vi "AAL Resample (const to Variable, complex single-channel).vi"(7 "reset? (True)":bool=TRUE, 8 "error in (no error)":errorcluster, 9 "config":T1={"timing jitter"=enum."Interpolation", "anti-aliasing?"=TRUE, "filter prototype"={"coefficients"=[], "factor"=1}} {"filter prototype"."coefficients" format="%.2f"}, 10 "time":dbl[](array[numeric]) format="%.2f", 11 "X":cdb[](array[numeric])) -> (0 "error out":errorcluster, 1 "offset":i64, 2 "time stamps":dbl[](array[numeric]) format="%.2f", 3 "Y":cdb[](array[numeric]) format="%.2f")   [LabVIEW 2017, in "NI_AALPro.lvlib"]
doc: "Perform an arbitrary resampling on the input signal."
uses:
  NI_AALPro.lvlib
  lvanlys.dll
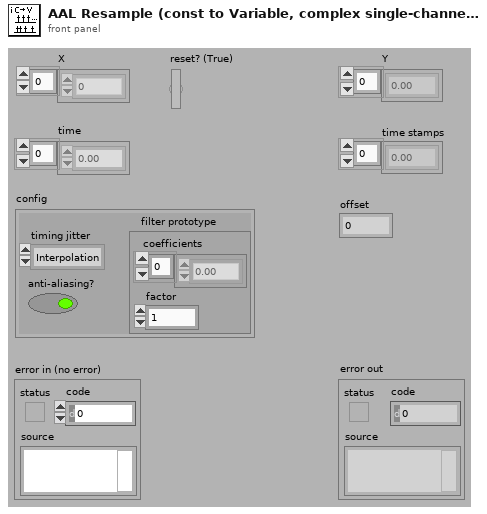
[diagram p1: front panel]
types:
  T1 = cluster{"timing jitter":enum32{"Interpolation", "Rounding"}, "anti-aliasing?":bool, "filter prototype":cluster{"coefficients":dbl[], "factor":i32}}
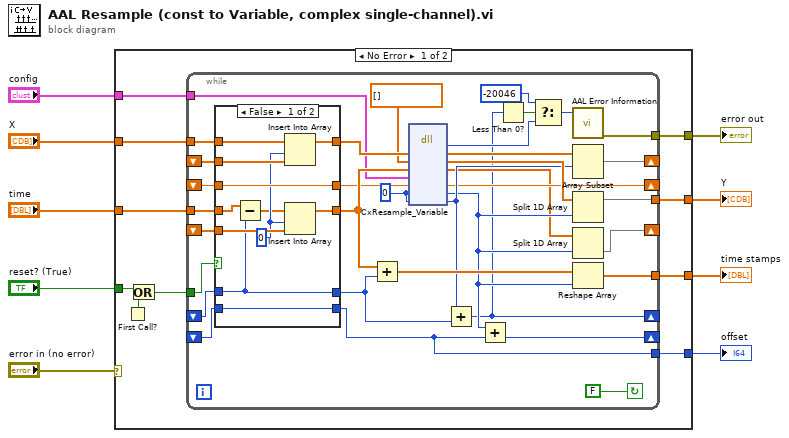
[diagram p0: block diagram]
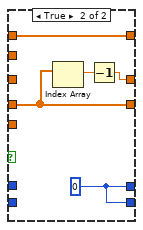
[diagram p2: hidden frame]
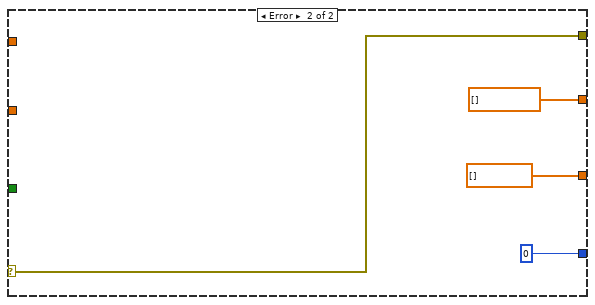
[diagram p3: hidden frame]
diagram:
  n1 = case shown="No Error" "error in (no error)" {
    selector: "error in (no error)" -> [_ w74]
    tunnel: "config" -> [w18 _]
    tunnel: "reset? (True)" -> [w17 _]
    tunnel: "time" -> [w11 _]
    tunnel: [w15 dbl[] []] -> w6
    tunnel: [w14 cdb[] []] -> w5
    tunnel: [w13 i64 0] -> w4
    tunnel: [w12 w74] -> w3
    tunnel: "X" -> [w10 _]
    frame No Error {
      n2 = First Call?() -> (First Call?: T/F=w19:bool)
      n3 = Or(x=w17, y=w19) -> (x .or. y?=w16:bool)
      n4 = while {
        tunnel: [w46] -> w14
        tunnel: [w39] -> w15
        shift-right: [w30] -> _
        shift-left: _ -> [w48]
        shift-right: [w54] -> _
        shift-left: _ -> [w49]
        tunnel: w10 -> [w52]
        tunnel: w11 -> [w50]
        shift-right: [w33] -> _
        shift-left: _ -> [w47]
        tunnel: w16 -> [w27]
        tunnel: w18 -> [w31]
        shift-right: [w20] -> _
        shift-left: _ -> [w26]
        tunnel: [w42] -> w13
        shift-right: [w41] -> _
        shift-left: _ -> [w43]
        tunnel: [w40] -> w12
        stop <- FALSE continue-if-true
        w37 = 0
        n5 = case shown="False" w27 {
          tunnel: [w64 w70] -> w51
          tunnel: w52 -> [w62 w70]
          tunnel: [w59 w69] -> w38
          tunnel: w50 -> [w58 w69]
          tunnel: [w65 w67] -> w32
          tunnel: w49 -> [w61 _]
          tunnel: w48 -> [w63 _]
          tunnel: w47 -> [w65 _]
          tunnel: w26 -> [w56 _]
          tunnel: [w56 w66] -> w25
          tunnel: w43 -> [w55 _]
          tunnel: [w55 w66] -> w42
          frame False {
            w60 = 0 ("Index")
            n6 = Subtract(x=w58, y=w56) -> (x-y=w57:dbl[])
            n7 = Insert Into Array(array=w62, index=w60, new element=w61) -> (w64:cdb[])
            n8 = Insert Into Array(array=w57, index=w60, new element=w63) -> (w59:dbl[])
          }
          frame True {
            w66 = i64 0
            n9 = Index Array(array=w69) -> (element=w68:dbl)  [unwired: 1 in]
            n10 = Decrement(x=w68) -> (x-1=w67:dbl)
          }
        }
        n11 = Add(x=w38, y=w25) -> (x+y=w45:dbl[])
        n12 = dll-call lib="C:/Program Files/National Instruments/LabVIEW 2017/resource/lvanlys.*" fn="CxResample_Variable"("X"=w51, "X"=cdb[] [], "timeH"=w38, "config"=w31, "last_sample_time"=w32, "out_len"=w37, "xLeftOverIdx"=w37) -> (w21:i32, "X"=w44:cdb[], "X"=w36:cdb[], "timeH"=w28:dbl[], "last_sample_time"=w33:dbl, "out_len"=w29:i32, "xLeftOverIdx"=w34:i32)  [unwired: 4 in, 2 out]
        n13 = Add(x=w34, y=w25) -> (x+y=w20:i64)
        n14 = Add(x=w29, y=w42) -> (x+y=w41:i64)
        n15 = Less Than 0?(x=w20) -> (x < 0?=w24:bool)
        n16 = Select(t=-20046 ("error"), s=w24, f=w21) -> (s? t:f=w22:i32)
        n17 = call "AAL Error Information.vi"("error code"=w22) -> ("error out"=w40:errorcluster)  [unwired: 10 in]
        n18 = Array Subset(array=w44, index=w34) -> (w54:cdb[])  [unwired: 1 in]
        n19 = Split 1D Array(array=w36, index=w29) -> (first subarray=w46:cdb[])  [unwired: 1 out]
        n20 = Split 1D Array(array=w28, index=w29) -> (second subarray=w30:dbl[])  [unwired: 1 out]
        n21 = Reshape Array(w45, w29) -> (w39:dbl[])
      }
    }
    frame Error {
    }
  }
  "time stamps" <- w6
  "Y" <- w5
  "offset" <- w4
  "error out" <- w3
